vi "DLL Connect and Read Config.vi"(8 "error in (no error)":errorcluster, 11 "Phasor Data Concentrator in":refnum<class "Phasor Data Concentrator.lvclass">) -> (0 "error out":errorcluster, 3 "Phasor Data Concentrator out":refnum<class "Phasor Data Concentrator.lvclass">)   [LabVIEW 2013, in "PMU Recorder Light.lvlib" / "Phasor Data Concentrator.lvclass"]
doc: "Calls the DLL class to connect to the PDC."
uses:
  Phasor Data Concentrator.lvclass
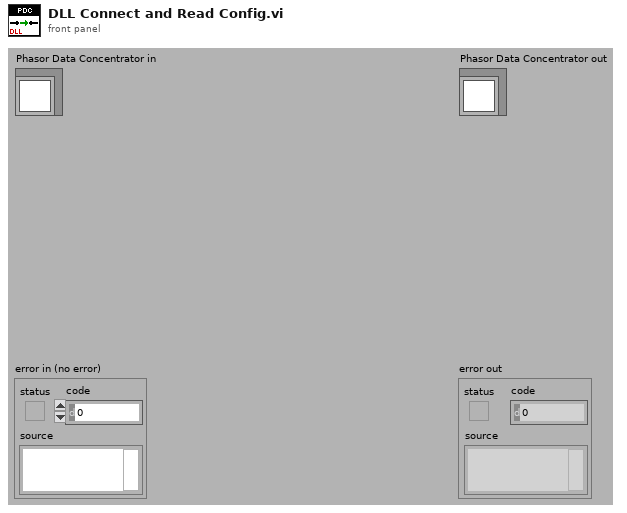
[diagram p1: front panel]
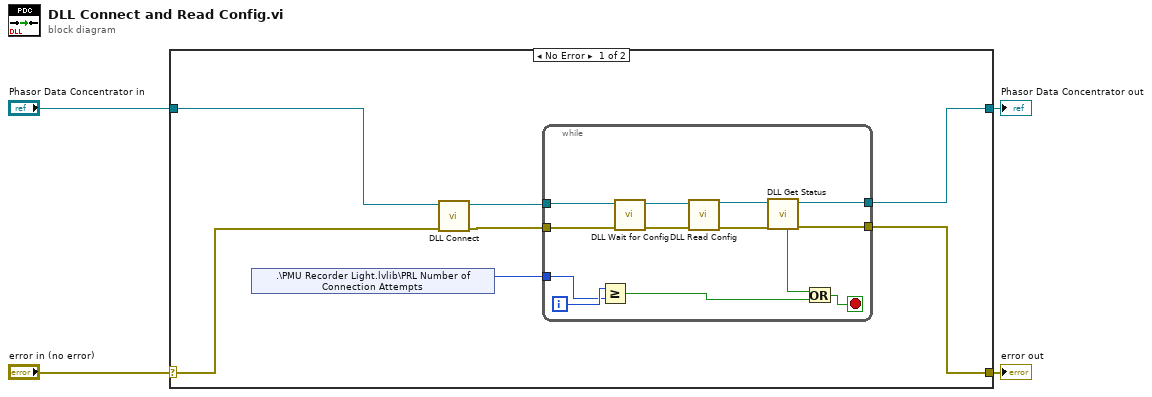
[diagram p0: block diagram]
diagram:
  n1 = case shown="No Error" "error in (no error)" {
    selector: "error in (no error)" -> [w5 w26]
    tunnel: [w11 w26] -> w3
    tunnel: [w10 w25] -> w1
    tunnel: "Phasor Data Concentrator in" -> [w6 w25]
    frame No Error {
      n2 = shared-variable ".\\PMU Recorder Light.lvlib\\PRL Number of Connection Attempts"() -> (w9:i32)  [unwired: 1 in, 1 out]
      n3 = call "DLL Connect.vi"("error in (no error)"=w5, "Phasor Data Concentrator in"=w6) -> ("error out"=w7:errorcluster, "Phasor Data Concentrator out"=w8:refnum<class "Phasor Data Concentrator.lvclass">)  [unwired: 8 in]
      n4 = while {
        tunnel: w8 -> [w13]
        tunnel: w7 -> [w12]
        tunnel: [w20] -> w11
        tunnel: [w19] -> w10
        tunnel: w9 -> [w17]
        i -> [w18]
        stop <- w14 stop-if-true
        n5 = Greater Or Equal?(x=w18, y=w17) -> (x >= y?=w15:bool)
        n6 = call "DLL Wait for Config.vi"("error in (no error)"=w12, "Phasor Data Concentrator in"=w13) -> ("error out"=w23:errorcluster, "Phasor Data Concentrator out"=w24:refnum<class "Phasor Data Concentrator.lvclass">)  [unwired: 8 in]
        n7 = call "DLL Read Config.vi"("error in (no error)"=w23, "Phasor Data Concentrator in"=w24) -> ("error out"=w21:errorcluster, "Phasor Data Concentrator out"=w22:refnum<class "Phasor Data Concentrator.lvclass">)  [unwired: 8 in]
        n8 = call "DLL Get Status.vi"("error in (no error)"=w21, "Phasor Data Concentrator in"=w22) -> ("error out"=w20:errorcluster, "Phasor Data Concentrator out"=w19:refnum<class "Phasor Data Concentrator.lvclass">, "Configuration Read OK"=w16:bool)  [unwired: 3 in, 4 out]
        n9 = Or(x=w16, y=w15) -> (x .or. y?=w14:bool)
      }
    }
    frame Error {
    }
  }
  "error out" <- w3
  "Phasor Data Concentrator out" <- w1
